vi "TCP Disconnect All Clients.vi"(8 "error in (no error)":errorcluster, 11 "TCP Server":refnum<class "JKI TCP Server.lvclass">) -> (0 "error out":errorcluster, 3 "TCP Server out":refnum<class "JKI TCP Server.lvclass">)   [LabVIEW 2020, in "JKI TCP Server.lvclass"]
uses:
  JKI TCP Server.lvclass
  JKI TCP Server.lvclass/JKI TCP Server.ctl
panel:
  # "Copyright © 2004-2008 JKI. All rights reserved.\n\nAuthor: Jim Kring [jim.kring@jameskring.com]\n\nThis library is provided \"AS IS\" ,WITHOUT WARRANTIES OR \nCONDITIONS OF ANY KIND, either express or implied.\n\nJames Kring, Inc. -- http://www.jameskring.com"
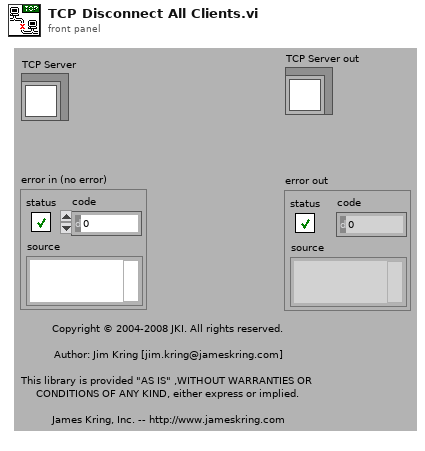
[diagram p1: front panel]
types:
  T1 = typedef "JKI TCP Server.lvclass/TCP Server Data.ctl" = cluster{"Listener Info":T2, "Connection Process VI RefNums":refnum<vi>[], "dup connection IDs (for quick search)":refnum<k5>[], "Connections":T3[], "Connection Handler VI Path":path, "Handler Is Reentrant?":bool, "TCP Handler Instance RefNums":T4[], "TCP Handler VI RefNum":T4, "No. Connections":u32, "Max Connections":u32, "server start time":u32, "Additional Data":variant}
  T2 = typedef "JKI TCP Server.lvclass/TCP Server Listener Info Cluster.ctl" = cluster{"listener ID":refnum<k5>, "net address":u32, "port":u16, "Listener Process VI Refnum":refnum<vi>}
  T3 = typedef "JKI TCP Server.lvclass/TCP Server Connection Info Cluster.ctl" = cluster{"connection ID":refnum<k5>, "Remote Address":string, "remote port":u16, "connection start time":u32}
  T4 = typedef "JKI TCP Server.lvclass/TCP Server Handler RefNum.ctl" = refnum<vi>
  T5 = cluster{"Connection Process VI Refnum":refnum<vi>, "TCP Handler VI RefNum":T4}
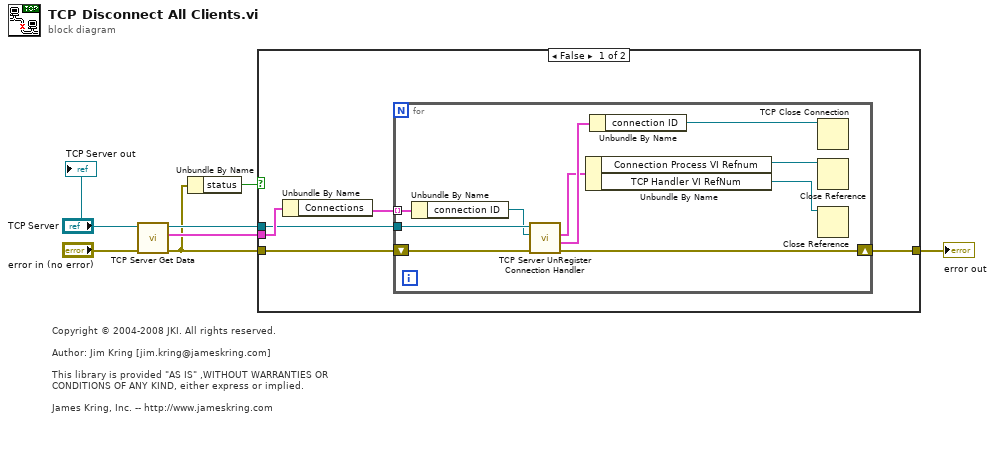
[diagram p0: block diagram]
diagram:
  # "Copyright © 2004-2008 JKI. All rights reserved.\n\nAuthor: Jim Kring [jim.kring@jameskring.com]\n\nThis library is provided \"AS IS\" ,WITHOUT WARRANTIES OR \nCONDITIONS OF ANY KIND, either express or implied.\n\nJames Kring, Inc. -- http://www.jameskring.com"
  n1 = call "TCP Server Get Data.vi"("error in (no error)"="error in (no error)", "RefNum"="TCP Server") -> ("error out"=w2:errorcluster, "Data out"=w6:T1, "dup RefNum"=w5:refnum<class "JKI TCP Server.lvclass">)  [unwired: 7 in]
  n2 = Unbundle By Name(w2) -> ("status"=w1:bool)
  n3 = case shown="False" w1 {
    tunnel: w6 -> [w12 _]
    tunnel: w5 -> [w11 _]
    tunnel: w2 -> [w10 w23]
    tunnel: [w9 w23] -> w4
    frame False {
      n4 = Unbundle By Name(w12) -> ("Connections"=w8:T3[])
      n5 = for {
        tunnel: w11 -> [w22]
        tunnel: w8 -> [w21] mode=indexing
        shift-right: [w19] -> w9
        shift-left: w10 -> [w20]
        n6 = Unbundle By Name(w21) -> ("connection ID"=w18:refnum<k5>)
        n7 = call "TCP Server UnRegister Connection Handler.vi"("error in (no error)"=w20, "connection ID"=w18, "TCP Server RefNum"=w22) -> ("error out"=w19:errorcluster, "Connection Info"=w17:T3, "VI References"=w16:T5)  [unwired: 6 in]
        n8 = Unbundle By Name(w16) -> ("Connection Process VI Refnum"=w14:refnum<vi>, "TCP Handler VI RefNum"=w13:T4)
        n9 = Unbundle By Name(w17) -> ("connection ID"=w15:refnum<k5>)
        n10 = TCP Close Connection(connection ID=w15) -> ()  [unwired: 2 in, 2 out]
        n11 = Close Reference(reference=w14) -> ()  [unwired: 1 in, 1 out]
        n12 = Close Reference(reference=w13) -> ()  [unwired: 1 in, 1 out]
      }
    }
    frame True {
      # "Error"
    }
  }
  "error out" <- w4
  "TCP Server out" <- "TCP Server"
